vi "Get Freq-Time Spectral Map (U8).vi"(7 "dB On (T)":bool=TRUE, 8 "error in (no error)":errorcluster, 10 "sampling frequency [Hz]":dbl=1.0 format="%.2f", 11 "RefNum in":T1) -> (0 "error out":errorcluster, 1 "quantization info":cluster{"offset":dbl, "multiplier":dbl} {"multiplier" format="%.2f"; "offset" format="%.2f"}, 2 "spectral map":u8[][](array[numeric]), 3 "RefNum out":T1, 4 "frequency scale":cluster{"offset":dbl, "multiplier":dbl} {"multiplier" format="%.2f"; "offset" format="%.2f"}, 5 "time scale":cluster{"offset":dbl, "multiplier":dbl} {"multiplier" format="%.2f"; "offset" format="%.2f"})   [LabVIEW 2017, in "SoundVib_Gabor.lvlib"]
doc: "Generates a frequency-time spectral map of the data block referenced by <B>RefNum in</B>. You can use this polymorphic VI to return <B>spectral map</B> as a 2D array of double-precision, floating-point numbers or a 2D array of 8-bit unsigned integers. You must manually select the polymorphic instance to use. Use the DBL instance to obtain more accurate data. Use the U8 instance to reduce memory usage when the VI displays data."
uses:
  <vilib>/addons/Sound and Vibration/Order Analysis/Gabor Order Tracking/SoundVib_Gabor.lvlib
  <vilib>/addons/Sound and Vibration/Order Analysis/Ref Gabor Order Tracking/GT RefNum.ctl
  <resource>/sndvib.dll
panel:
  # "Get Freq-Time Spectral Map (U8)"
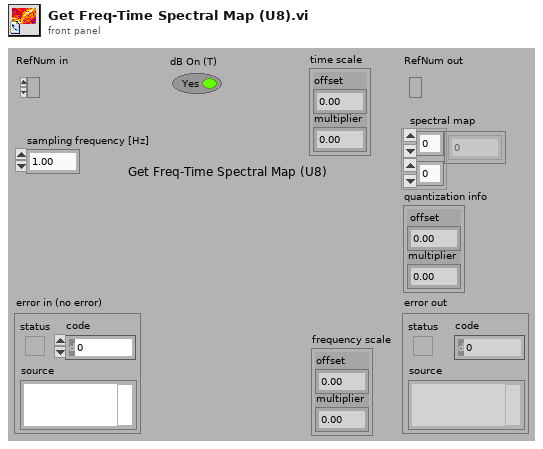
[diagram p1: front panel]
types:
  T1 = typedef "SoundVib_Gabor.lvlib/GT RefNum.ctl" = refnum<k1>
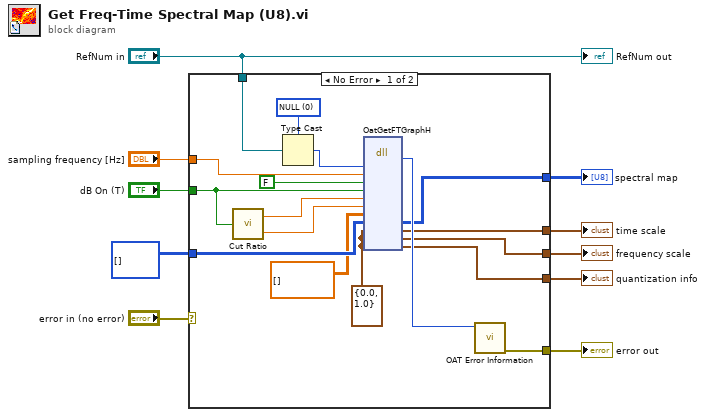
[diagram p0: block diagram]
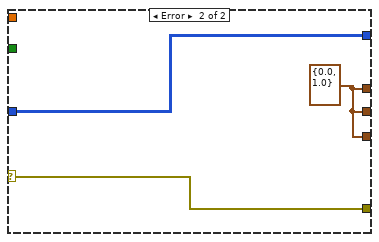
[diagram p2: hidden frame]
diagram:
  n1 = case shown="No Error" "error in (no error)" {
    selector: "error in (no error)" -> [_ w30]
    tunnel: [w27 w30] -> w7
    tunnel: "RefNum in" -> [w23 _]
    tunnel: "dB On (T)" -> [w13 _]
    tunnel: [w22 w29] -> w6
    tunnel: u8[][] [] ("Graph") -> [w17 w29]
    tunnel: [w18 w28] -> w4
    tunnel: [w20 w28] -> w3
    tunnel: [w21 w28] -> w2
    tunnel: "sampling frequency [Hz]" -> [w11 _]
    frame No Error {
      w19 = cluster{"Z Min":dbl, "Z Step":dbl} {"Z Min"=0.0, "Z Step"=1.0}
      w26 = u32 0 items=["NULL"]
      n2 = call <vilib>:"Cut Ratio.vi"("dB On (T)"=w13) -> ("UpperCutRatio"=w14:dbl, "LowerCutRatio"=w15:dbl)
      n3 = Type Cast(type=w26, x=w23) -> (*(type *) &x=w25:u32)
      n4 = dll-call lib="C:/Program Files (x86)/National Instruments/LabVIEW 2017/resource/sndvib.*" fn="OatGetFTGraphH"("Ref In"=w25, "Fs"=w11, "bGetDBL"=FALSE, "bLogZ"=w13, "UpperCutRatio"=w14, "LowerCutRatio"=w15, "DBLGraph"=dbl[][] [], "U8Graph"=w17, "XScale"=w19, "YScale"=w19, "ZScale"=w19) -> ("return type"=w24:i32, "U8Graph"=w22:u8[][], "XScale"=w21:cluster{"Z Min":dbl, "Z Step":dbl}, "YScale"=w20:cluster{"Z Min":dbl, "Z Step":dbl}, "ZScale"=w18:cluster{"Z Min":dbl, "Z Step":dbl})  [unwired: 10 in, 2 out]
      n5 = call <vilib>:"OAT Error Information.vi"("error code"=w24) -> ("error out"=w27:errorcluster)  [unwired: 6 in]
    }
    frame Error {
      w28 = cluster{"Z Min":dbl, "Z Step":dbl} {"Z Min"=0.0, "Z Step"=1.0}
    }
  }
  "error out" <- w7
  "spectral map" <- w6
  "quantization info" <- w4
  "time scale" <- w2
  "frequency scale" <- w3
  "RefNum out" <- "RefNum in"
